vi "Example TCP Send Image.vi"() -> ()   [LabVIEW 2016]
panel:
  out "Success?":bool
  out "Error":errorcluster
  in  "Remote Port Number":u16=30000
  in  "Remote IP Address":string="131.111.45.97"
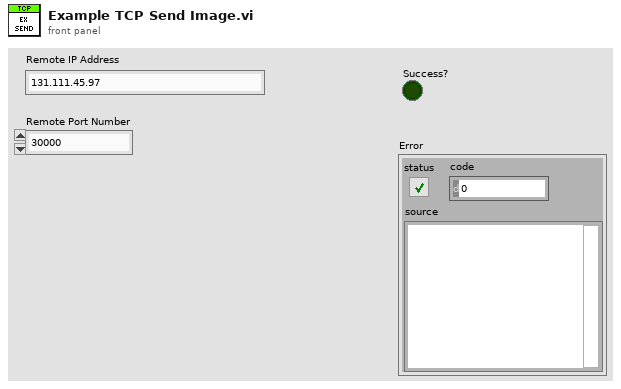
[diagram p1: front panel]
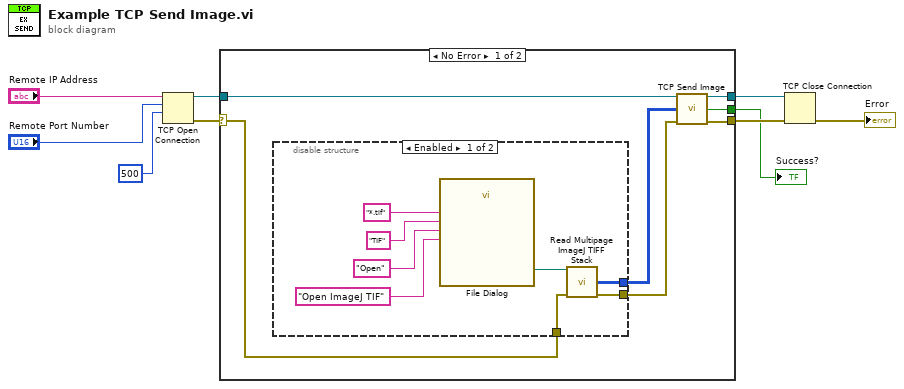
[diagram p0: block diagram]
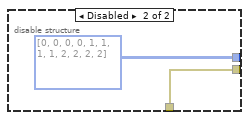
[diagram p2: hidden frame]
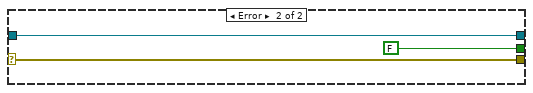
[diagram p3: hidden frame]
diagram:
  n1 = TCP Open Connection(address="Remote IP Address", remote port or service name="Remote Port Number", timeout ms (60000)=500) -> (connection ID=w5:refnum<k5>, error out=w6:errorcluster)  [unwired: 2 in]
  n2 = case shown="No Error" w6 {
    selector: w6 -> [w11 w28]
    tunnel: w5 -> [w16 w29]
    tunnel: [w15 w29] -> w4
    tunnel: [w14 w28] -> w3
    tunnel: [w12 FALSE ("Success?")] -> w1
    frame No Error {
      n3 = disable-structure shown="Enabled" {
        disable-tunnel: [w20 u16[][][] [[[0, 0], [0, 0]], [[1, 1], [1, 1]], [[2, 2], [2, 2]]]] -> w13
        disable-tunnel: w11 -> [w18 w25]
        disable-tunnel: [w17 w25] -> w10
        frame Enabled {
          n4 = call "File Dialog"("prompt"="Open ImageJ TIF", "button label"="Open", "pattern (all files)"="*.tif", "pattern label"="TIF") -> ("selected path"=w19:path)  [unwired: 8 in, 3 out]
          n5 = call "Read Multipage ImageJ TIFF Stack.vi"("ImageJ Tif Path"=w19, "Error In"=w18) -> ("U16 Stack"=w20:u16[][][], "Error Out"=w17:errorcluster)  [unwired: 9 in, 3 out]
        }
        frame Disabled {
        }
      }
      n6 = call "TCP Send Image.vi"("Connection ID"=w16, "Image Stack (U16)"=w13, "Error In"=w10) -> ("Connection ID Out"=w15:refnum<k5>, "Success?"=w12:bool, "Error Out"=w14:errorcluster)  [unwired: 10 in]
    }
    frame Error {
    }
  }
  "Success?" <- w1
  n7 = TCP Close Connection(connection ID=w4, error in (no error)=w3) -> (error out=→"Error":errorcluster)  [unwired: 1 in, 1 out]
